vi "Read Measurement (Efficiency Power Analysis).vi"(0 "VISA resource name":refnum<visa-resource-name>, 5 "Efficiency Measurement Type (0: Efficiency)":i32(ring) items=["Efficiency", "Input Power", "Output Power"], 11 "error in (no error)":errorcluster) -> (4 "VISA resource name out":refnum<visa-resource-name>, 6 "Efficiency Measurement":dbl, 15 "error out":errorcluster)   [LabVIEW 2019, in "Agilent 2000 3000 X-Series.lvlib"]
doc: "Returns the measurement of a efficiency power analysis.\n\n<B>Note(s):</B>\nUse <B>Configure Power Analysis (Efficiency).vi</B> to apply a power analysis."
uses:
  Agilent 2000 3000 X-Series.lvlib
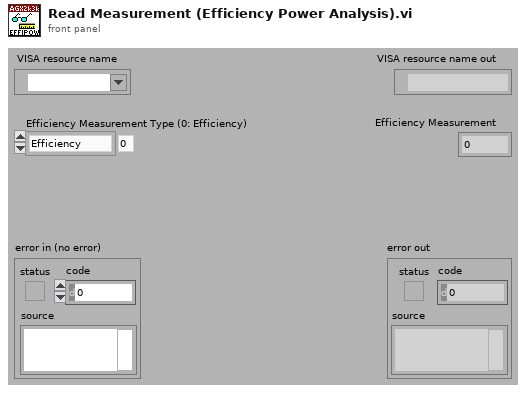
[diagram p1: front panel]
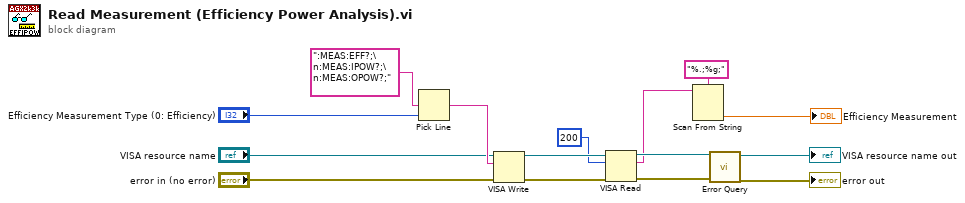
[diagram p0: block diagram]
diagram:
  n1 = Pick Line(multi-line string=":MEAS:EFF?;\n:MEAS:IPOW?;\n:MEAS:OPOW?;", line index="Efficiency Measurement Type (0: Efficiency)") -> (output string=w13:string)  [unwired: 1 out]
  n2 = VISA Write(VISA resource name="VISA resource name", write buffer=w13, error in (no error)="error in (no error)") -> (VISA resource name out=w8:refnum<visa-resource-name>, error out=w7:errorcluster)  [unwired: 1 out]
  n3 = VISA Read(VISA resource name=w8, byte count=u32 200, error in (no error)=w7) -> (VISA resource name out=w5:refnum<visa-resource-name>, read buffer=w2:string, error out=w4:errorcluster)  [unwired: 1 out]
  n4 = Scan From String(format string="%.;%g;", input string=w2) -> (output 1=→"Efficiency Measurement":dbl)  [unwired: 2 in, 4 out]
  n5 = call "Error Query.vi"("error in (no error)"=w4, "VISA resource name"=w5) -> ("error out"=→"error out":errorcluster, "VISA resource name out"=→"VISA resource name out":refnum<visa-resource-name>)  [unwired: 8 out]
